vi "Global - UI Streams and Variables.vi"() -> ()   [LabVIEW 2017]
uses:
  Support/Message Queue/Message Cluster.ctl
  Controls/Variable References.ctl
  Controls/Manual Control.ctl
  Support/Message Queue/Message Queue.lvlib
panel:
  in  "Variable References":T1
  in  "UI Command Stream":refnum<k21>
  in  "RT Message Stream":refnum<k21>
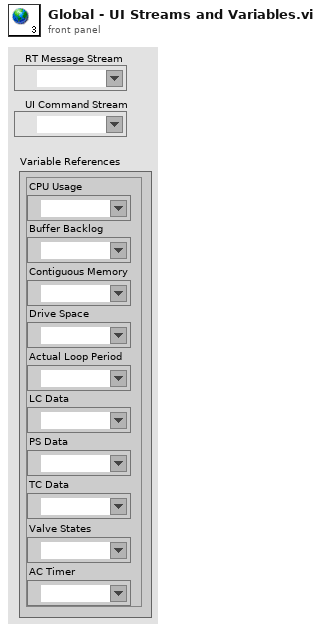
[diagram p1: front panel]
types:
  T1 = typedef "Variable References.ctl" = cluster{"CPU Usage":refnum<k21>, "Buffer Backlog":refnum<k21>, "Contiguous Memory":refnum<k21>, "Drive Space":refnum<k21>, "Actual Loop Period":refnum<k21>, "LC Data":refnum<k21>, "PS Data":refnum<k21>, "TC Data":refnum<k21>, "Valve States":refnum<k21>, "AC Timer":refnum<k21>}
diagram:
